vi "sub_ExecutionTime.vi"(7 "State":T1, 8 "error in":errorcluster caption="에러 입력") -> (0 "error out":errorcluster caption="에러 출력", 3 "Elapsed Time (sec)":dbl format="%#.2g")   [LabVIEW 2017]
uses:
  Control/Time.ctl
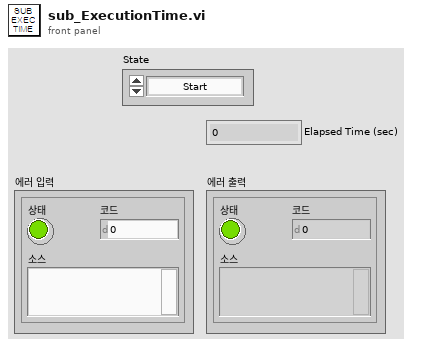
[diagram p1: front panel]
types:
  T1 = typedef "Time.ctl" = enum16{"Start", "End"}
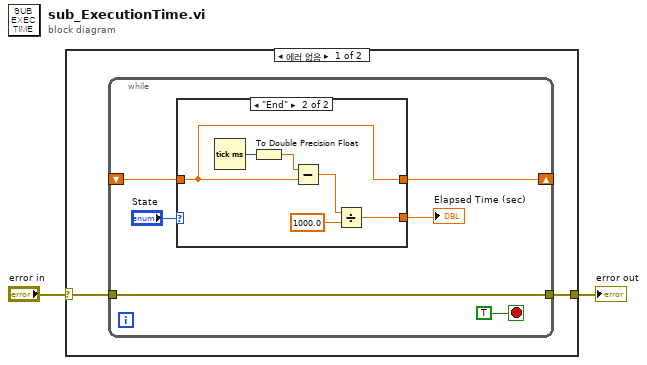
[diagram p0: block diagram]
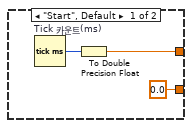
[diagram p2: hidden frame]
diagram:
  n1 = case shown="에러 없음" "error in" {
    selector: "error in" -> [w4 w20]
    tunnel: [w3 w20] -> w1
    frame No Error {
      n2 = while {
        tunnel: w4 -> [w10]
        tunnel: [w10] -> w3
        shift-right: [w6] -> _
        shift-left: _ -> [w7]
        stop <- TRUE stop-if-true
        n3 = case shown="\"End\"" "State" {
          tunnel: w7 -> [_ w14]
          tunnel: [w12 w14] -> w6
          tunnel: [0.0 w15] -> w5
          frame "Start", Default {
            n4 = Tick Count (ms) "Tick 카운트(ms)"() -> (millisecond timer value=w13:u32)
            n5 = To Double Precision Float(number=w13) -> (double precision float=w12:dbl)
          }
          frame "End" {
            n6 = Tick Count (ms)() -> (millisecond timer value=w19:u32)
            n7 = To Double Precision Float(number=w19) -> (double precision float=w18:dbl)
            n8 = Subtract(x=w18, y=w14) -> (x-y=w17:dbl)
            n9 = Divide(x=w17, y=1000.0) -> (x/y=w15:dbl)
          }
        }
        "Elapsed Time (sec)" <- w5
      }
    }
    frame Error {
    }
  }
  "error out" <- w1
